vi "Create Gradient Color Ramp V2.vi"(11 "Color Array":u32[](array[colorbox])=[16711680, 16448250, 16860]) -> (0 "Horizontal Color Ramp":i32[][](graph), 1 "Vertical Color Ramp":i32[][](graph), 3 "Color Table":u32[](array[numeric]))   [LabVIEW 2013]
panel:
  out "1 Pix H - Color Box Array":u32[](array[colorbox])
  out "1 Pix W - Color Box Array":u32[](array[colorbox])
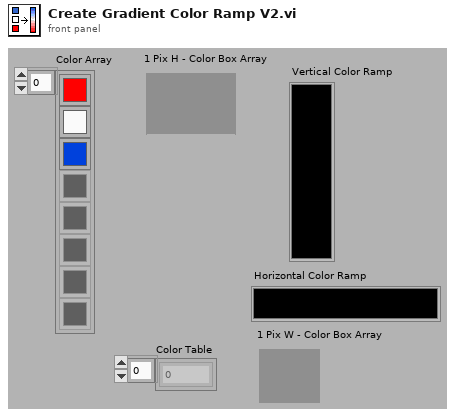
[diagram p1: front panel]
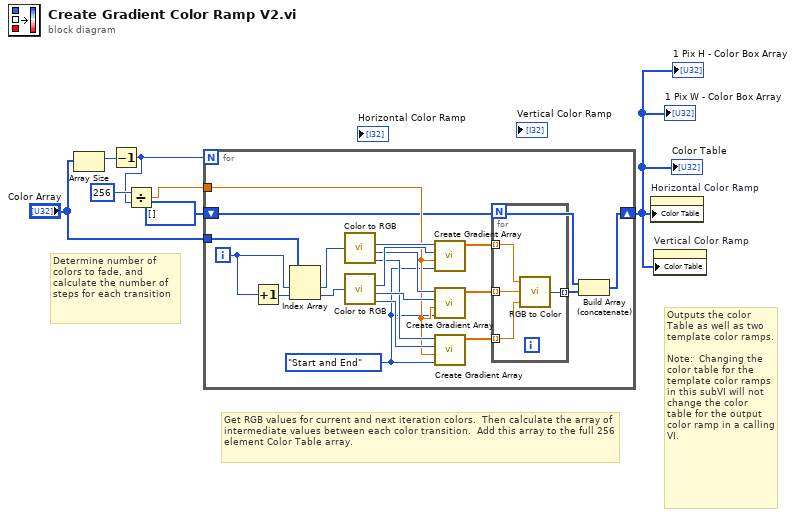
[diagram p0: block diagram]
diagram:
  # "Outputs the color Table as well as two template color ramps.  \n\nNote:  Changing the color table for the template color ramps in this subVI will not change the color table for the output color ramp in a calling VI."
  # "Get RGB values for current and next iteration colors.  Then calculate the array of intermediate values between each color transition.  Add this array to the full 256 element Color Table array."
  # "Determine number of colors to fade, and calculate the number of steps for each transition"
  n1 = Array Size(array="Color Array") -> (size(s)=w3:i32)
  n2 = Decrement(x=w3) -> (x-1=w2:i32)
  n3 = Divide(x=256, y=w2) -> (x/y=w6:dbl)
  n4 = for {
    N: w2 -> [_]
    tunnel: "Color Array" -> [w26]
    tunnel: w6 -> [w15]
    shift-right: [w8] -> w1
    shift-left: u32[] [] -> [w9]
    i -> [w25]
    w14 = enum16{"Start", "End", "Start and End", "None"}."Start and End" ("Values to Include")
    n5 = Increment(x=w25) -> (x+1=w24:i32)
    n6 = Index Array(array=w26, index #1=w25, index #2=w24) -> (element #1=w23:u32, element #2=w22:u32)
    n7 = call <vilib>:"Color to RGB.vi"("Color"=w23) -> ("R"=w21:u8, "G"=w19:u8, "B"=w17:u8)  [unwired: 1 out]
    n8 = call <vilib>:"Color to RGB.vi"("Color"=w22) -> ("R"=w20:u8, "G"=w18:u8, "B"=w16:u8)  [unwired: 1 out]
    n9 = call "Create Gradient Array.vi"("Values to Include"=w14, "Array Length"=w15, "End Value"=w20, "Start Value"=w21) -> ("Output Array"=w13:dbl[])  [unwired: 7 in]
    n10 = call "Create Gradient Array.vi"("Values to Include"=w14, "Array Length"=w15, "End Value"=w18, "Start Value"=w19) -> ("Output Array"=w12:dbl[])  [unwired: 7 in]
    n11 = call "Create Gradient Array.vi"("Values to Include"=w14, "Array Length"=w15, "End Value"=w16, "Start Value"=w17) -> ("Output Array"=w11:dbl[])  [unwired: 7 in]
    n12 = for {
      tunnel: w13 -> [w29] mode=indexing
      tunnel: w12 -> [w30] mode=indexing
      tunnel: w11 -> [w28] mode=indexing
      tunnel: [w27] -> w10 mode=indexing
      n13 = call <vilib>:"RGB to Color.vi"("B"=w28, "G"=w30, "R"=w29) -> ("Color"=w27:u32)
    }
    n14 = Build Array (concatenate)(w9, w10) -> (w8:u32[])
  }
  "Color Table" <- w1
  "1 Pix W - Color Box Array" <- w1
  "1 Pix H - Color Box Array" <- w1
  n15 = property on="Horizontal Color Ramp" class="IntGraph (strict)"("Color Table"=w1) -> ()  [unwired: 2 in, 2 out]
  n16 = property on="Vertical Color Ramp" class="IntGraph (strict)"("Color Table"=w1) -> ()  [unwired: 2 in, 2 out]
